vi "Swift.constructor.vi"(0 "name":string, 2 "data in":string, 5 "error in(no error)":errorcluster) -> (14 "i ref out":refnum<vi>, 16 "data out":string, 19 "error out":errorcluster)   [LabVIEW 2014, in "Swift.lvlib"]
doc: "This is the constructor of a class.\n\nLicense Agreement for this software:\n\nCopyright (C)\nGesellschaft für Schwerionenforschung, GSI\nPlanckstr. 1\n64291 Darmstadt\nGermany\n\nContact: D.Beck@gsi.de \n\nThis program is free software; you can redistribute it and/or modify it under the terms of the \nGNU General Public License as published by the Free Software Foundation; either version 2 of \nthe license, or (at your option) any later version.\n\nThis program is distributed in the hope that it will be useful, but WITHOUT ANY WARRANTY; \nwithout even the implied warranty of MERCHANTABILITY or FITNESS FOR A PARTICULAR PURPOSE. See the GNU General License for more details (http://www.gnu.org).\n\nGesellschaft für Schwerionenforschung, GSI\nPlanckstr. 1, 64291 Darmstadt, Germany\nFor all questions and ideas contact: M.Richter@gsi.de, H.Brand@gsi.de or D.Beck@gsi.de.\nLast update: 16-JUN-2004"
uses:
  Swift.lvlib
  CSCore/CSSystem/CoreLib/CoreLib.string 2 byte array.vi
  CSCore/BaseProcess/BaseProcess.lvlib
  CSCore/CSSystem/CSSystemLib/CSSystemLib.lvlib
  CSCore/CSSystem/CoreLib/CoreLib.lvlib
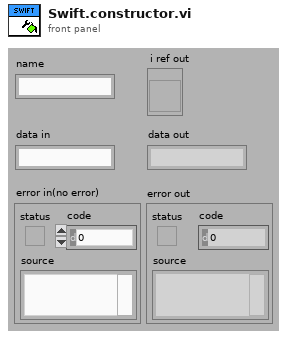
[diagram p1: front panel]
types:
  T1 = enum16{"SetAttribute", "GetAttribute", "CreateAttribute", "DestroyAttribute", "DestroyAllAtributes"}
  T2 = typedef "BaseProcess.lvlib/BaseProcess.i attribute.ctl" = cluster{"EventStatus":string, "EventError":i32, "PresetEvtWatchD":i32, "PresetPdcWatchD":i32, "EventTimeout":i32, "PeriodicInterval":i32, "Interface":string[], "Address":string[], "Special":string[], "PeriodicError":i32, "PeriodicStatus":string, "SuperProc":string, "Descriptors":T3[], "CaseRef":refnum<vi>, "PdcRef":refnum<vi>, "Thread Ref":refnum<vi>, "eventErrorID":i32, "eventStatusID":i32, "periodicErrorID":i32, "periodicStatusID":i32, "pdcCtrID":i32}
  T3 = typedef "BaseProcess.lvlib/BaseProcess.descriptor definition.ctl" = cluster{"selector":string, "descriptor":T4}
  T4 = typedef "BaseProcess.lvlib/BaseProcess.descriptor string definition.ctl" = string
  T5 = typedef "Swift.lvlib/Swift.i attribute.ctl" = cluster{"SWIFT Frequency Generator":string}
  T6 = typedef "CoreDefs.rawDataType.ctl" = i8[]
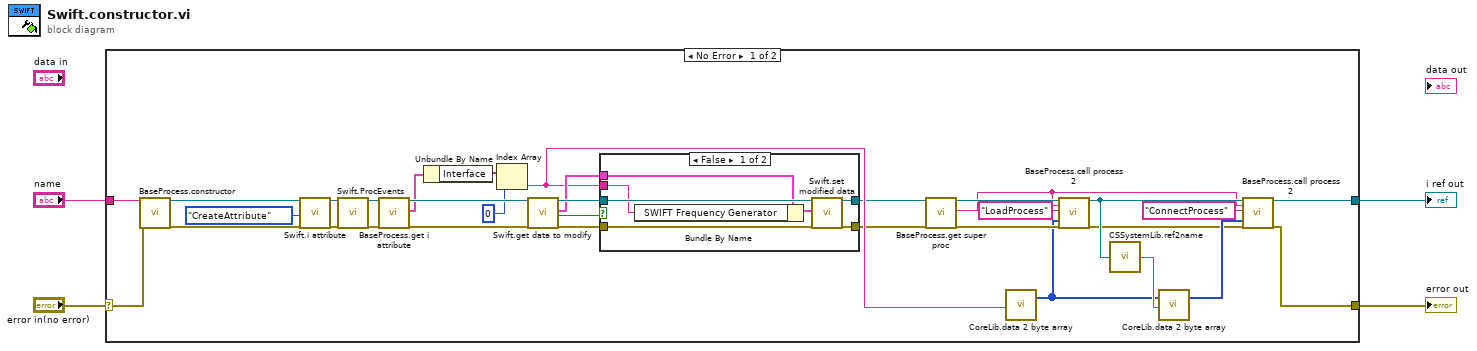
[diagram p0: block diagram]
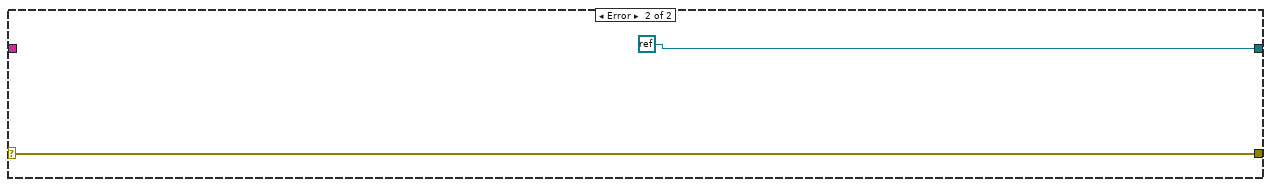
[diagram p3: hidden frame]
diagram:
  n1 = case shown="No Error" "error in(no error)" {
    selector: "error in(no error)" -> [w31 w48]
    tunnel: "name" -> [w34 _]
    tunnel: [w7 refnum<k0> refnum] -> w3
    tunnel: [w6 w48] -> w2
    frame No Error {
      n2 = call "BaseProcess.constructor.vi"("name"=w34, "error in (no error)"=w31) -> ("i ref out"=w37:refnum<vi>, "error out"=w36:errorcluster)  [unwired: 15 in, 1 out]
      n3 = call "Swift.i attribute.vi"("VI Refnum"=w37, "Action"=T1."CreateAttribute", "error in (no error)"=w36) -> ("VI Refnum out"=w33:refnum<vi>, "error out"=w32:errorcluster)  [unwired: 14 in, 1 out]
      n4 = call "Swift.ProcEvents.vi"("i ref in"=w33, "error in"=w32) -> ("i ref out"=w26:refnum<vi>, "error out"=w24:errorcluster)  [unwired: 16 in]
      n5 = call "BaseProcess.get i attribute.vi"("i ref in"=w26, "error in (no error)"=w24) -> ("i ref out"=w25:refnum<vi>, "i attribute"=w22:T2, "error out"=w23:errorcluster)  [unwired: 15 in]
      n6 = Unbundle By Name(w22) -> ("Interface"=w21:string[])
      n7 = Index Array(array=w21, index=0) -> (element=w9:string)
      n8 = call "Swift.get data to modify.vi"("i ref in"=w25, "error in (no error)"=w23) -> ("i ref out"=w29:refnum<vi>, "CLASS.i attribute out"=w27:T5, "timed out"=w30:bool, "error out"=w28:errorcluster)  [unwired: 14 in]
      n9 = case shown="False" w30 {
        tunnel: [w44 w45] -> w5
        tunnel: [w43 w46] -> w8
        tunnel: w29 -> [w42 w46]
        tunnel: w28 -> [w41 w45]
        tunnel: w27 -> [w40 _]
        tunnel: w9 -> [w38 _]
        frame False {
          n10 = Bundle By Name(cluster=w40, "SWIFT Frequency Generator"=w38) -> (w39:T5)
          n11 = call "Swift.set modified data.vi"("i ref in"=w42, "i attribute"=w39, "error in (no error)"=w41) -> ("i ref out"=w43:refnum<vi>, "error out"=w44:errorcluster)  [unwired: 15 in]
        }
        frame True {
        }
      }
      n12 = call "BaseProcess.get super proc.vi"("i ref in"=w8, "error in (no error)"=w5) -> ("i ref out"=w16:refnum<vi>, "SuperProc"=w12:string, "error out"=w14:errorcluster)  [unwired: 15 in]
      n13 = call-poly "CoreLib.data 2 byte array.vi"("string"=w9) -> ("byteArray out"=w10:T6)  [unwired: 18 in]
      n14 = call "BaseProcess.call process 2.vi"("i ref in"=w16, "Object"=w12, "Selector"="LoadProcess", "Data"=w10, "error in (no error)"=w14) -> ("i ref out"=w15:refnum<vi>, "error out"=w13:errorcluster)  [unwired: 13 in]
      n15 = call "CSSystemLib.ref2name.vi"("obj refnum"=w15) -> ("name"=w18:string)
      n16 = call-poly "CoreLib.data 2 byte array.vi"("byteArray"=w10, "string"=w18) -> ("byteArray out"=w17:T6)  [unwired: 17 in]
      n17 = call "BaseProcess.call process 2.vi"("i ref in"=w15, "Object"=w12, "Selector"="ConnectProcess", "Data"=w17, "error in (no error)"=w13) -> ("i ref out"=w7:refnum<vi>, "error out"=w6:errorcluster)  [unwired: 13 in]
    }
    frame Error {
    }
  }
  "i ref out" <- w3
  "error out" <- w2
